vi "시스템 실행.vi"() -> ()   [LabVIEW 2014]
panel:
  out "Ping Result":string
  in  "Ping":bool
  in  "컴퓨터 IP":string
  in  "화면 전환":bool
  in  "문자표":bool
  in  "소리조절":bool
  in  "Stop":bool
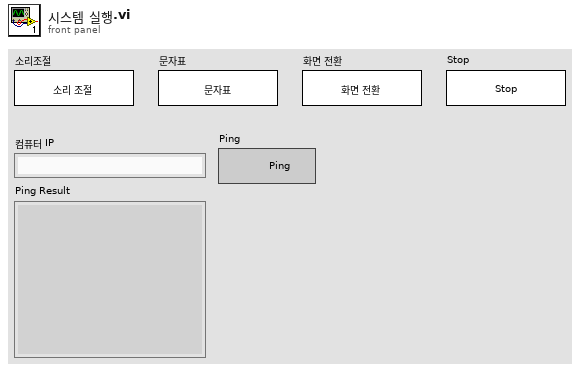
[diagram p1: front panel]
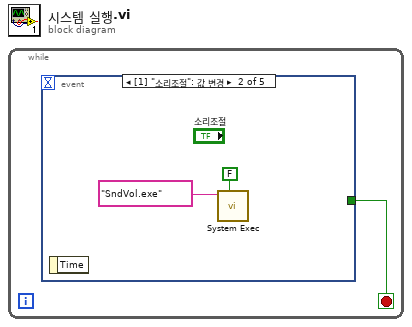
[diagram p0: block diagram]
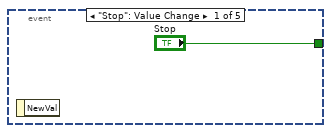
[diagram p2: hidden frame]
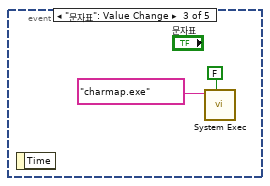
[diagram p3: hidden frame]
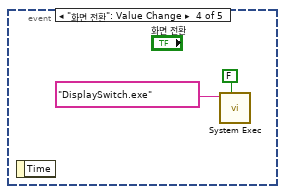
[diagram p4: hidden frame]
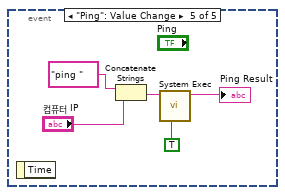
[diagram p5: hidden frame]
diagram:
  n1 = while {
    stop <- w1 stop-if-true
    n2 = event shown="[1] \"소리조절\": 값 변경" {
      selector: _ -> [_ _ _ _ _]
      dyn-events: _ -> [_ _ _ _ _]
      timeout: _ -> [_ _ _ _ _]
      tunnel: ["Stop" _ _ _ _] -> w1
      event "Stop": Value Change {
        n3 = event-data() -> ()  [unwired: 1 in, 1 out]
      }
      event "소리조절": Value Change {
        n4 = event-data() -> ()  [unwired: 1 in, 1 out]
        n5 = call <vilib>:"System Exec.vi"("wait until completion? (T)"=FALSE, "command line"="SndVol.exe") -> ()  [unwired: 6 in, 4 out]
      }
      event "문자표": Value Change {
        n6 = event-data() -> ()  [unwired: 1 in, 1 out]
        n7 = call <vilib>:"System Exec.vi"("wait until completion? (T)"=FALSE, "command line"="charmap.exe") -> ()  [unwired: 6 in, 4 out]
      }
      event "화면 전환": Value Change {
        n8 = event-data() -> ()  [unwired: 1 in, 1 out]
        n9 = call <vilib>:"System Exec.vi"("wait until completion? (T)"=FALSE, "command line"="DisplaySwitch.exe") -> ()  [unwired: 6 in, 4 out]
      }
      event "Ping": Value Change {
        n10 = event-data() -> ()  [unwired: 1 in, 1 out]
        n11 = Concatenate Strings("ping " ("command line"), "컴퓨터 IP") -> (w11:string)
        n12 = call <vilib>:"System Exec.vi"("run minimized? (F)"=TRUE, "command line"=w11) -> ("standard output"=→"Ping Result":string)  [unwired: 6 in, 3 out]
      }
    }
  }
